vi "Destroy.vi"(8 "error in (no error)":errorcluster, 11 "TopLevel in":refnum<class "IO.lvclass">) -> (0 "error out":errorcluster, 3 "TopLevel out":refnum<class "IO.lvclass">)   [LabVIEW 2022 SP3, in "IO.lvclass"]
uses:
  IO.lvclass
  IO.lvclass/IO.ctl
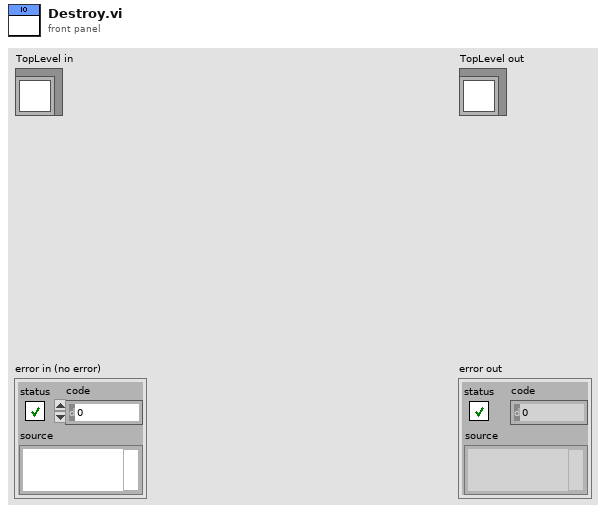
[diagram p1: front panel]
types:
  T1 = typedef "IO.lvclass/Private Data.ctl" = cluster{"UserEvents":T2, "All Dependencies":cluster{"Class References":refnum<class>[], "Class Names":string[]}, "Status":T3}
  T2 = typedef "IO.lvclass/UserEvents.ctl" = cluster{"API Incoming Event":refnum<user-event>, "API Executed Event":refnum<user-event>, "API Return Event":refnum<user-event>, "Status Changed Event":refnum<user-event>}
  T3 = typedef "IO.lvclass/Status Cluster.ctl" = cluster{"Device Data":variant, "Ordered ICP1-DO Channels":T4[], "Ordered ICP2-DI Channels":T5[], "Ordered ICP2-DO Channels":T6[], "Ordered ICP1-AI Channels":T7[], "Ordered ICP1-AO Channels":T8[], "Ordered ICP2-AO Channels":T9[]}
  T4 = typedef "IO.lvclass/ICP1-D0 Channel Names.ctl" = enum16{"None", "Meniscus Pressure Reg PWR - R1", "Meniscus Pressure Reg PWR - R2", "Meniscus Pressure Reg PWR - R3", "Meniscus Pressure Reg PWR - R4", "Meniscus Pressure Reg PWR - R5", "Meniscus Pressure Reg PWR - R6", "Clear Stage Alarm", "Servo ON", "Purge Valve Open - R1", "Purge Valve Open - R2", "Purge Valve Open - R3", "Purge Valve Open - R4", "Purge Valve Open - R5", "Purge Valve Open - R6"}
  T5 = typedef "IO.lvclass/ICP2-DI Channel Names.ctl" = enum16{"None", "SW - Ink Valve - R1", "SW - Ink Valve - R2", "SW - Ink Valve - R3", "SW - Ink Valve - R4", "SW - Ink Valve - R5", "SW - Ink Valve - R6", "SW - COVER INPUT SIDE", "SW - COVER OUTPUT SIDE", "SW - Purge - R1", "SW - Purge - R2", "SW - Purge - R3", "SW - Purge - R4", "SW - Purge - R5", "SW - Purge - R6"}
  T6 = typedef "IO.lvclass/ICP2-DO Channel Names.ctl" = enum16{"None", "Meniscus Valve Open - R1", "Meniscus Valve Open - R2", "Meniscus Valve Open - R3", "Meniscus Valve Open - R4", "Meniscus Valve Open - R5", "Meniscus Valve Open - R6", "Ink Flow Valve Open - R1", "Ink Flow Valve Open - R2", "Ink Flow Valve Open - R3", "Ink Flow Valve Open - R4", "Ink Flow Valve Open - R5", "Ink Flow Valve Open - R6", "SW_LED - Ink Valve - R1", "SW_LED - Ink Valve - R2", "SW_LED - Ink Valve - R3", "Recirc Pump On - R1", "Recirc Pump On - R2", "Recirc Pump On - R3", "Recirc Pump On - R4", "Recirc Pump On - R5", "Recirc Pump On - R6", "SW_LED - Ink Valve - R4", "SW_LED - Ink Valve - R5", "SW_LED - Ink Valve - R6"}
  T7 = typedef "IO.lvclass/ICP1-AI Channel Names.ctl" = enum16{"None", "Meniscus Pressure Read - R1", "Meniscus Pressure Read - R2", "Meniscus Pressure Read - R3", "Meniscus Pressure Read - R4", "Meniscus Pressure Read - R5", "Meniscus Pressure Read - R6", "Meniscus Pressure Set - R1", "Meniscus Pressure Set - R2", "Meniscus Pressure Set - R3", "Meniscus Pressure Set - R4", "Meniscus Pressure Set - R5", "Meniscus Pressure Set - R6"}
  T8 = typedef "IO.lvclass/ICP1-AO Channel Names.ctl" = enum16{"None", "Meniscus Pressure Set - R1", "Meniscus Pressure Set - R2", "Meniscus Pressure Set - R3", "Meniscus Pressure Set - R4", "Meniscus Pressure Set - R5", "Meniscus Pressure Set - R6", "Meniscus Vac Pump Speed"}
  T9 = typedef "IO.lvclass/ICP2-AO Channel Names.ctl" = enum16{"None", "Recirc Pump Flow Set - R1", "Recirc Pump Flow Set - R2", "Recirc Pump Flow Set - R3", "Recirc Pump Flow Set - R4", "Recirc Pump Flow Set - R5", "Recirc Pump Flow Set - R6"}
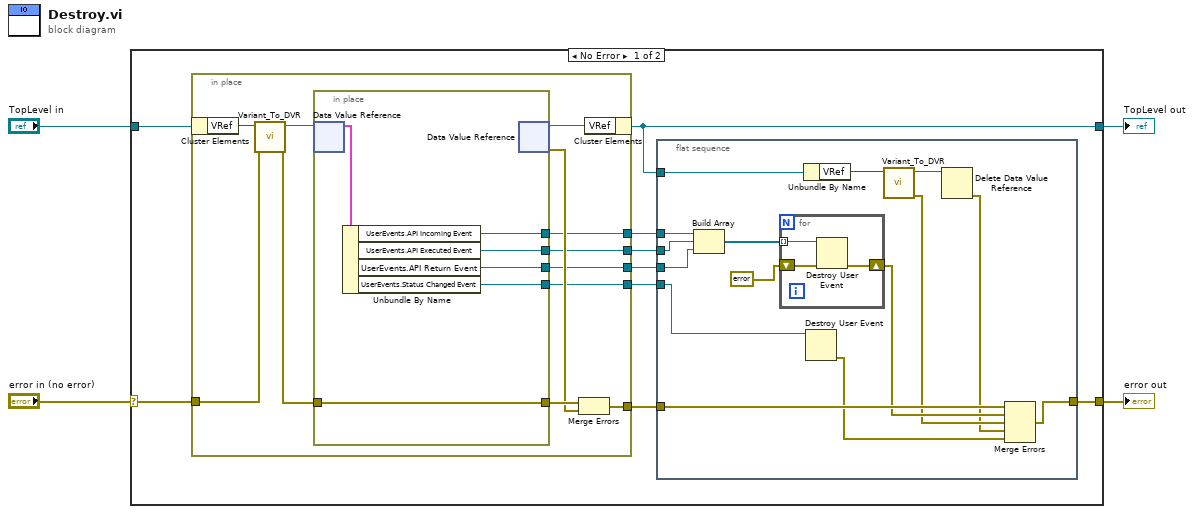
[diagram p0: block diagram]
diagram:
  n1 = case shown="No Error" "error in (no error)" {
    selector: "error in (no error)" -> [w12 w51]
    tunnel: [w8 w51] -> w3
    tunnel: [w9 w50] -> w1
    tunnel: "TopLevel in" -> [w13 w50]
    frame No Error {
      n2 = in-place {
        in-place-border: w12 -> [w40]
        in-place-border: [w36] -> w10
        in-place-border: [w35] -> w11
        in-place-border: [w34] -> w7
        in-place-border: [w33] -> w6
        in-place-border: [w32] -> w5
        n3 = in-place-cluster #1(w13) -> ("VRef"=w43:variant)
        n4 = call "Variant_To_DVR.vi"("error in (no error)"=w40, "Variant"=w43) -> ("error out"=w39:errorcluster, "DVR"=w42:refnum<data-value>)  [unwired: 8 in]
        n5 = in-place {
          in-place-border: [w48] -> w35
          in-place-border: w39 -> [w47]
          in-place-border: [w47] -> w38
          in-place-border: [w46] -> w34
          in-place-border: [w45] -> w33
          in-place-border: [w44] -> w32
          n6 = in-place-dvr #2(w42) -> (w49:T1)  [unwired: 1 out]
          n7 = Unbundle By Name(w49) -> ("UserEvents.API Incoming Event"=w48:refnum<user-event>, "UserEvents.API Executed Event"=w46:refnum<user-event>, "UserEvents.API Return Event"=w45:refnum<user-event>, "UserEvents.Status Changed Event"=w44:refnum<user-event>)
          n8 = in-place-dvr #2() -> (w41:refnum<data-value>, w37:errorcluster)  [unwired: 1 in]
        }
        n9 = Merge Errors(w38, w37) -> (w36:errorcluster)
        n10 = in-place-cluster #1("VRef"=w41) -> (w9:refnum<class "IO.lvclass">)
      }
      n11 = flat-sequence {
        tunnel: w11 -> [w19]
        tunnel: w10 -> [w24]
        tunnel: w9 -> [w27]
        tunnel: [w22] -> w8
        tunnel: w7 -> [w18]
        tunnel: w6 -> [w17]
        tunnel: w5 -> [w15]
        frame #0 {
          n12 = Build Array(w19, w18, w17) -> (w16:refnum<user-event>[])
          n13 = for {
            tunnel: w16 -> [w31] mode=indexing
            shift-right: [w30] -> w23
            shift-left: errorcluster {"status"=FALSE, "code"=0, "source"=""} ("error constant") -> [w29]
            n14 = Destroy User Event(user event=w31, error in=w29) -> (error out=w30:errorcluster)
          }
          n15 = Unbundle By Name(w27) -> ("VRef"=w26:variant)
          n16 = Destroy User Event(user event=w15) -> (error out=w14:errorcluster)  [unwired: 1 in]
          n17 = call "Variant_To_DVR.vi"("Variant"=w26) -> ("error out"=w21:errorcluster, "DVR"=w25:refnum<data-value>)  [unwired: 9 in]
          n18 = Delete Data Value Reference(data value reference=w25) -> (error out=w20:errorcluster)  [unwired: 1 in, 1 out]
          n19 = Merge Errors(w24, w23, w21, w20, w14) -> (w22:errorcluster)
        }
      }
    }
    frame Error {
    }
  }
  "error out" <- w3
  "TopLevel out" <- w1
